vi "RightClickType.vi"(10 "Mod":T2, 11 "MouseDownState":T3) -> (3 "RightClickType":T1)   [LabVIEW 2021, in "RocketPlot.lvlib"]
uses:
  RocketPlot.lvlib
  TypeDefs/MouseDownState.ctl
  TypeDefs/RightClickCache PlatMod.ctl
  TypeDefs/RightClickType.ctl
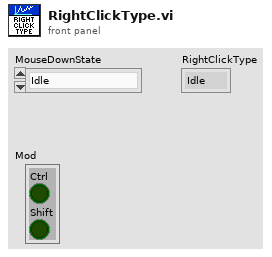
[diagram p1: front panel]
types:
  T1 = typedef "RocketPlot.lvlib/RightClickType.ctl" = enum16{"Idle", "Delta", "SliceAvg", "Identify"}
  T2 = typedef "RocketPlot.lvlib/RightClickCache PlatMod.ctl" = cluster{"Ctrl":bool, "Shift":bool}
  T3 = typedef "RocketPlot.lvlib/MouseDownState.ctl" = enum16{"Idle", "Pan", "Zoom", "Zoom-Post", "RightClick"}
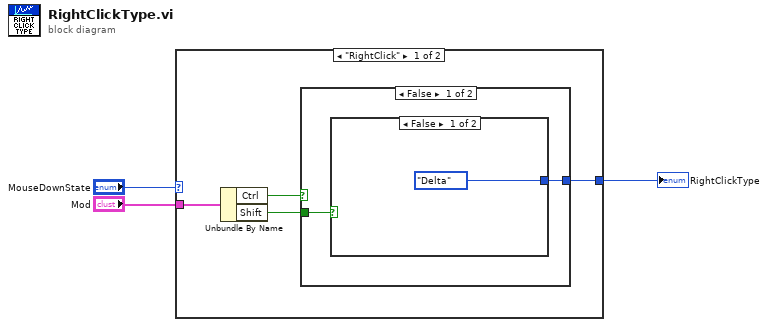
[diagram p0: block diagram]
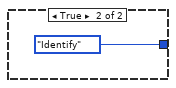
[diagram p2: hidden frame]
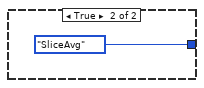
[diagram p3: hidden frame]
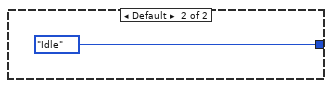
[diagram p4: hidden frame]
diagram:
  n1 = case shown="\"RightClick\"" "MouseDownState" {
    tunnel: [w5 RightClickType."Idle" ("Enum")] -> w2
    tunnel: "Mod" -> [w7 _]
    frame "RightClick" {
      n2 = Unbundle By Name(w7) -> ("Ctrl"=w6:bool, "Shift"=w4:bool)
      n3 = case shown="False" w6 {
        tunnel: [w8 RightClickType."SliceAvg" ("Enum")] -> w5
        tunnel: w4 -> [w9 _]
        frame False {
          n4 = case shown="False" w9 {
            tunnel: [RightClickType."Delta" ("Enum") RightClickType."Identify" ("Enum")] -> w8
            frame False {
            }
            frame True {
            }
          }
        }
        frame True {
        }
      }
    }
    frame Default {
    }
  }
  "RightClickType" <- w2
